vi "P3_3_Elipse.vi"() -> ()   [LabVIEW 2020]
panel:
  out "XY Graph":cluster{dbl[], dbl[]}(graph)
  in  "B":dbl
  in  "A":dbl
  out "Array":dbl[](array[numeric])
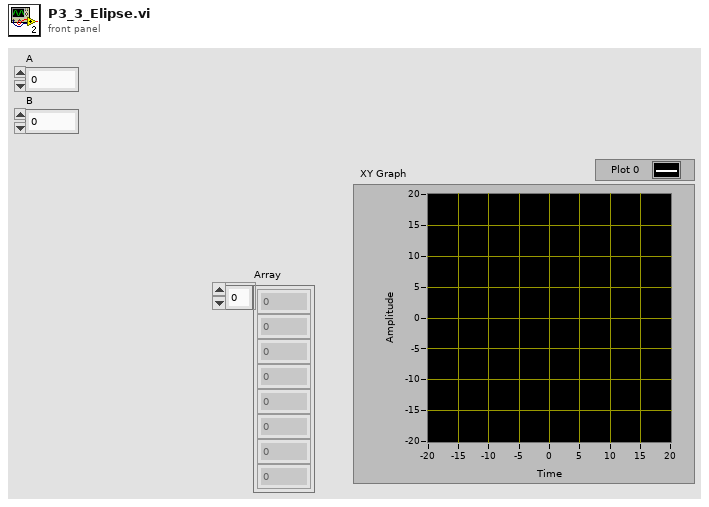
[diagram p1: front panel]
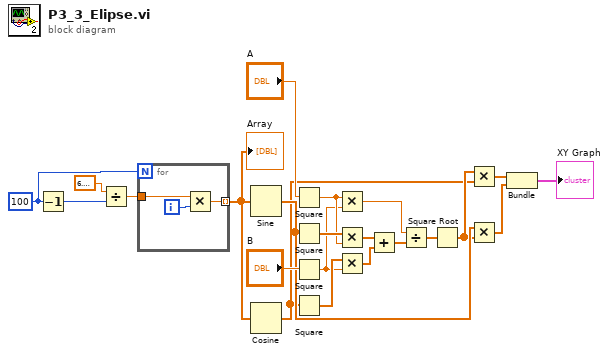
[diagram p0: block diagram]
diagram:
  w22 = 100
  n1 = Decrement(x=w22) -> (x-1=w21:i32)
  n2 = Divide(x=6.283185307179586, y=w21) -> (x/y=w19:dbl)
  n3 = for {
    N: w22 -> [_]
    tunnel: w19 -> [w24]
    tunnel: [w23] -> w18 mode=indexing
    i -> [w25]
    n4 = Multiply(x=w24, y=w25) -> (x*y=w23:dbl)
  }
  "Array" <- w18
  n5 = Sine(x=w18) -> (sin(x)=w6:dbl[])
  n6 = Cosine(x=w18) -> (cos(x)=w4:dbl[])
  n7 = Square(x="A") -> (x^2=w13:dbl)
  n8 = Square(x=w6) -> (x^2=w14:dbl[])
  n9 = Square(x="B") -> (x^2=w12:dbl)
  n10 = Square(x=w4) -> (x^2=w15:dbl[])
  n11 = Multiply(x=w13, y=w12) -> (x*y=w9:dbl)
  n12 = Multiply(x=w14, y=w13) -> (x*y=w11:dbl[])
  n13 = Multiply(x=w15, y=w12) -> (x*y=w10:dbl[])
  n14 = Add(x=w11, y=w10) -> (x+y=w8:dbl[])
  n15 = Divide(x=w9, y=w8) -> (x/y=w7:dbl[])
  n16 = Square Root(x=w7) -> (sqrt(x)=w5:dbl[])
  n17 = Multiply(x=w5, y=w4) -> (x*y=w3:dbl[])
  n18 = Multiply(x=w6, y=w5) -> (x*y=w2:dbl[])
  n19 = Bundle "Bundle"(w3, w2) -> (→"XY Graph":cluster{dbl[], dbl[]})  [unwired: 1 in]
